vi "PFI-28000-Utils_Trim String.vi"(2 "location (both)":T1 items=["both", "start of string", "end of string"], 5 "String":string) -> (6 "Trimmed String":string)   [LabVIEW 2017, in "PFI-28000-Utils.lvlib"]
uses:
  PFI-28000-Utils.lvlib
  <vilib>/Utility/error.llb/whitespace.ctl
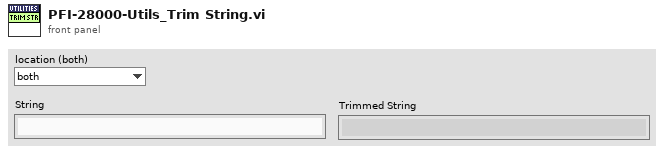
[diagram p1: front panel]
types:
  T1 = typedef "whitespace.ctl" = u16
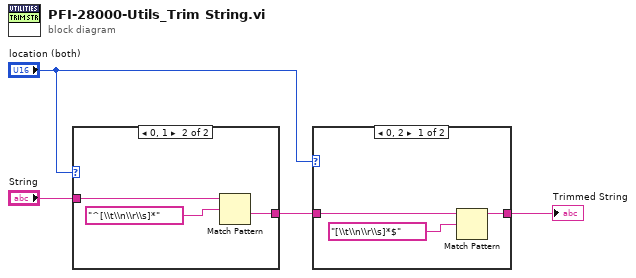
[diagram p0: block diagram]
diagram:
  n1 = case shown="0, 1" "location (both)" {
    tunnel: [w5 w8] -> w4
    tunnel: "String" -> [w5 w6]
    frame Default {
    }
    frame 0, 1 {
      n2 = Match Pattern(string=w6, regular expression="^[\\t\\n\\r\\s]*") -> (after substring=w8:string)  [unwired: 1 in, 3 out]
    }
  }
  n3 = case shown="0, 2" "location (both)" {
    tunnel: [w11 w12] -> w1
    tunnel: w4 -> [w10 w12]
    frame 0, 2 {
      n4 = Match Pattern(string=w10, regular expression="[\\t\\n\\r\\s]*$") -> (before substring=w11:string)  [unwired: 1 in, 3 out]
    }
    frame Default {
    }
  }
  "Trimmed String" <- w1
